vi "LVPortUpdateBoundProperty.vi"(0 "pID":string, 5 "Property":string, 7 "Properties":string[](array[string])) -> ()   [LabVIEW 2017]
uses:
  <userlib>/_OpenG.lib/dictionary/dictionary.llb/Dictionary Key Value Pair Cluster__ogtk.ctl
  <userlib>/_OpenG.lib/dictionary/dictionary.llb/Dictionary Update (by scalar value)__ogtk.vi
panel:
  in  "Update? (t)":bool=TRUE
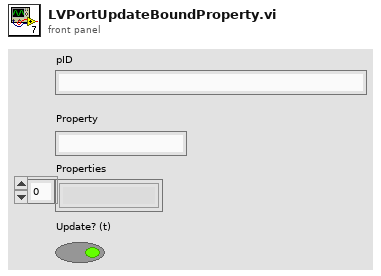
[diagram p1: front panel]
types:
  T1 = typedef "Dictionary Object RefNum__ogtk.ctl" = refnum<k1>
  T2 = typedef "Dictionary Key Value Pair Cluster__ogtk.ctl" = cluster{"key":variant, "value":variant}
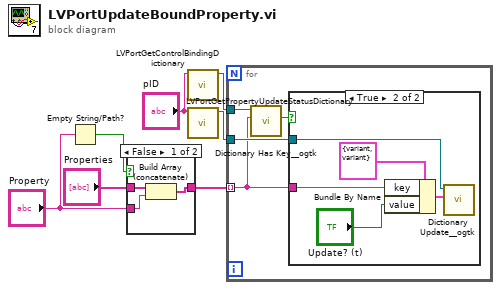
[diagram p0: block diagram]
diagram:
  n1 = Empty String/Path?(string/path="Property") -> (empty?=w6:bool)
  n2 = case shown="False" w6 {
    tunnel: "Properties" -> [w10 w11]
    tunnel: [w8 w11] -> w3
    tunnel: "Property" -> [w9 _]
    frame False {
      n3 = Build Array (concatenate)(w10, w9) -> (w8:string[])
    }
    frame True {
    }
  }
  n4 = call "LVPortGetControlBindingDictionary.vi"("pID"="pID") -> ("Refnum out"=w1:T1)  [unwired: 10 in]
  n5 = call "LVPortGetPropertyUpdateStatusDictionary.vi"("pID"="pID") -> ("Refnum out"=w2:T1)  [unwired: 10 in]
  n6 = for {
    tunnel: w3 -> [w12] mode=indexing
    tunnel: w2 -> [w13]
    tunnel: w1 -> [w15]
    n7 = call <userlib>:"Dictionary Has Key__ogtk.vi"("key"=w12, "dictionary"=w15) -> ("Has Key?"=w14:bool)  [unwired: 7 in, 2 out]
    n8 = case shown="True" w14 {
      tunnel: w13 -> [_ w20]
      tunnel: w12 -> [_ w17]
      frame False {
      }
      frame True {
        n9 = Bundle By Name(cluster=T2 {"key"=variant, "value"=variant} ("key-value"), "key"=w17, "value"="Update? (t)") -> (w18:T2)
        n10 = call-poly <userlib>:"Dictionary Update__ogtk.vi"("key-value"=w18, "dictionary"=w20) -> ()  [unwired: 7 in, 3 out]
      }
    }
  }
